vi "interactive_tester.vi"() -> ()   [LabVIEW 2024]
doc: "This VI can perform a measurement with the stimuli set by the Load control.\nBy pressing Update Values the measurement is performed."
uses:
  ctl_loads_enum.ctl
  ctl_stimuli_cluster.ctl
panel:
  out "Vdrop =":dbl
  out "Device OK":bool
  in  "btn_test_device":bool
  in  "DAQmx Device Name":tag="Dev1"
  out "Measurement in progress...":bool
  in  "btn_stop":bool
  in  "btn_update":bool
  out "Pin =":dbl
  out "Iout =":dbl
  in  "Load =":T1=enum."10Ohm"
  out "Efficiency =":dbl
  out "Pout =":dbl
  out "Vout =":dbl
  in  "Rsense =":dbl
  out "Iin =":dbl
  out "Vin =":dbl
  out "RL4":bool=TRUE
  out "RL3":bool=TRUE
  out "RL2":bool=TRUE
  out "RL1":bool=TRUE
  # "V"
  # "A"
  # "9 V"
  # "A"
  # "LM317"
  # "W"
  # "W"
  # "Ohm"
  # "V"
  # "DC-DC converter"
  # "V"
  # "%"
  # "Test the device connection before start measuring"
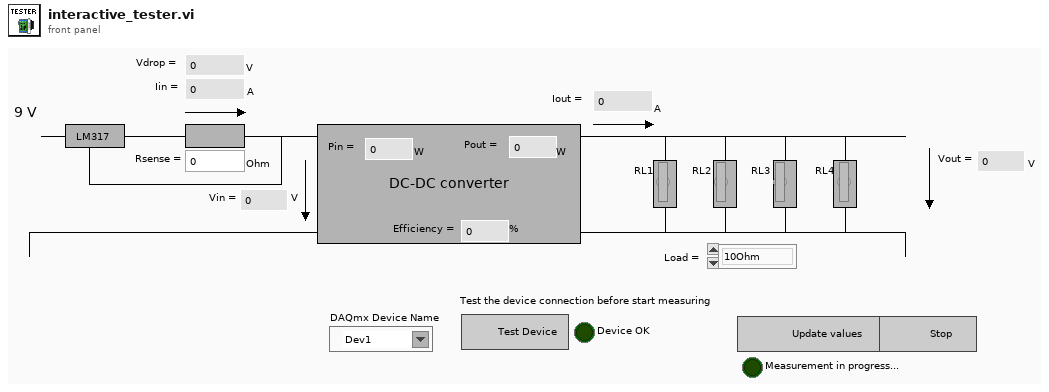
[diagram p1: front panel]
types:
  T1 = typedef "ctl_loads_enum.ctl" = enum16{"NO LOAD", "10Ohm", "6.8Ohm", "4.7Ohm", "3.3Ohm", "2.4Ohm", "1.6Ohm", "1.3Ohm"}
  T2 = typedef "ctl_stimuli_cluster.ctl" = cluster{"Load":T1, "Rsense Value":dbl}
  T3 = typedef "ctl_load_set_cluster.ctl" = cluster{"Resistor 1":bool, "Resistor 2":bool, "Resistor 3":bool, "Resistor 4":bool}
  T4 = typedef "ctl_test_outputs_cluster.ctl" = cluster{"Output V avg":dbl, "Output V ampl":dbl, "Input Current":dbl, "Output Current":dbl, "Efficiency %":dbl, "Input V avg":dbl, "Input Power":dbl, "Output Power":dbl, "Rsense Vdrop":dbl}
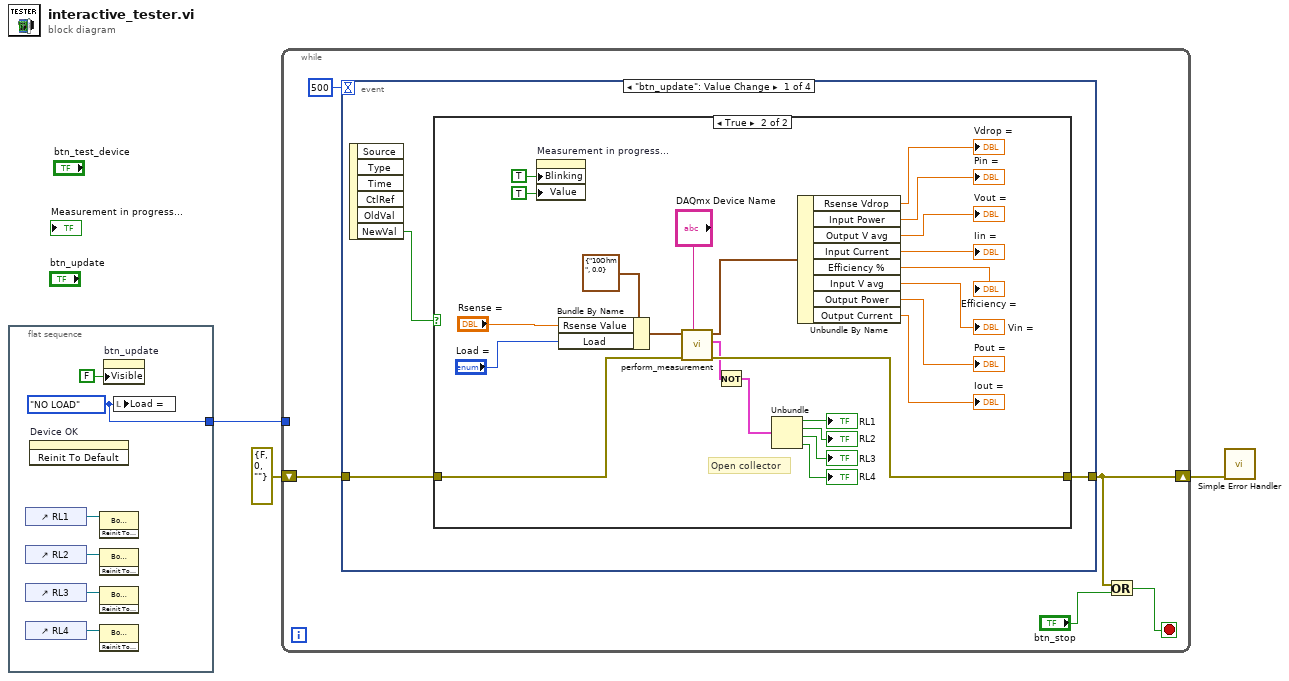
[diagram p0: block diagram]
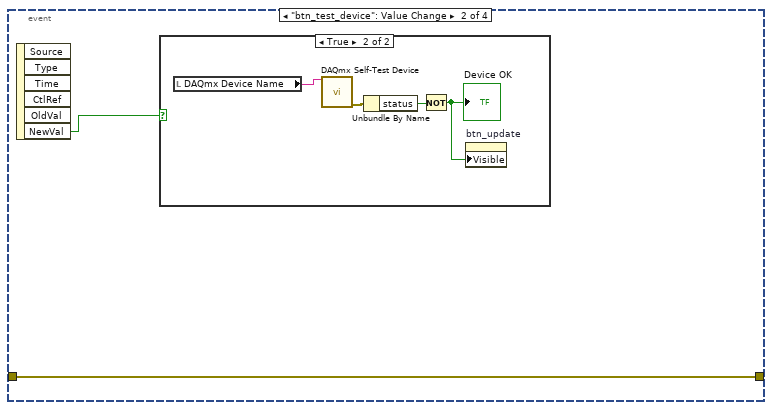
[diagram p3: hidden frame]
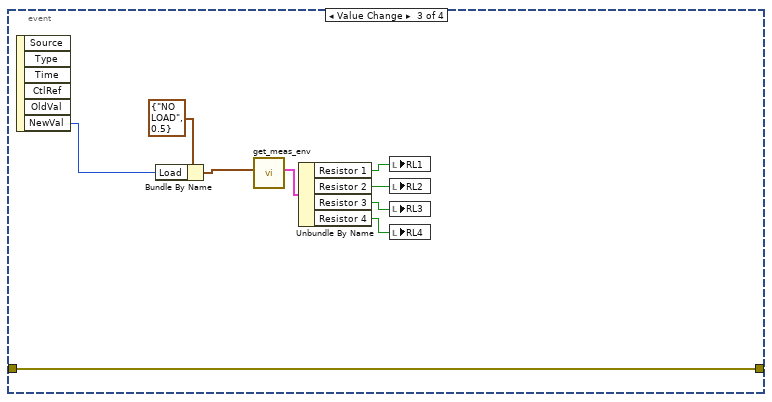
[diagram p5: hidden frame]
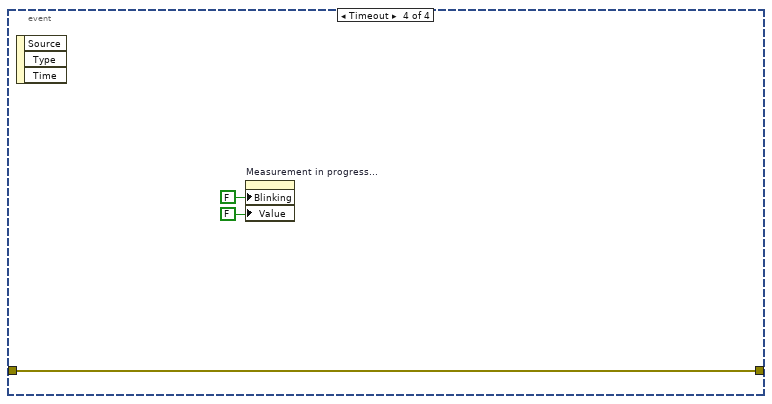
[diagram p6: hidden frame]
diagram:
  n1 = flat-sequence {
    tunnel: [w9] -> w3
    frame #0 {
      w9 = ctl_loads_enum."NO LOAD" ("Load =")
      n2 = control-ref of="RL1"() -> (w7:refnum<vi>)
      n3 = control-ref of="RL2"() -> (w6:refnum<vi>)
      n4 = control-ref of="RL3"() -> (w5:refnum<vi>)
      n5 = control-ref of="RL4"() -> (w4:refnum<vi>)
      n6 = invoke on="Device OK" class="Bool (strict)" method="Reinit To Default"() -> ()  [unwired: 3 in, 3 out]
      n7 = invoke class="Bool (strict)" method="Reinit To Default"(reference=w7) -> ()  [unwired: 2 in, 3 out]
      n8 = invoke class="Bool (strict)" method="Reinit To Default"(reference=w6) -> ()  [unwired: 2 in, 3 out]
      n9 = invoke class="Bool (strict)" method="Reinit To Default"(reference=w5) -> ()  [unwired: 2 in, 3 out]
      n10 = invoke class="Bool (strict)" method="Reinit To Default"(reference=w4) -> ()  [unwired: 2 in, 3 out]
      n11 = property on="btn_update" class="Bool (strict)"("Visible"=FALSE) -> ()  [unwired: 2 in, 2 out]
      n12 = local write "Load ="(w9) -> ()
    }
  }
  n13 = while {
    tunnel: w3 -> [_]
    shift-right: [w11] -> w1
    shift-left: errorcluster {"status"=FALSE, "code"=0, "source"=""} ("error out") -> [w13]
    stop <- w10 stop-if-true
    n14 = event shown="[0] \"btn_update\": Value Change" {
      selector: _ -> [_ _ _ _]
      dyn-events: _ -> [_ _ _ _]
      timeout: 500 -> [_ _ _ _]
      tunnel: [w16 w44 w49 w58] -> w11
      tunnel: w13 -> [w15 w44 w49 w58]
      event "btn_update": Value Change {
        n15 = event-data() -> ("NewVal"=w17:bool)  [unwired: 1 in, 5 out]
        n16 = case shown="True" w17 {
          tunnel: [w18 w24] -> w16
          tunnel: w15 -> [w18 w23]
          frame False {
          }
          frame True {
            # "Open collector"
            n17 = property on="Measurement in progress..." class="Bool (strict)"("Blinking"=TRUE, "Value"=TRUE ("Measurement in progress...")) -> ()  [unwired: 2 in, 2 out]
            n18 = Bundle By Name(cluster=T2 {"Load"=enum."10Ohm", "Rsense Value"=0.0} ("Stimuli"), "Rsense Value"="Rsense =", "Load"="Load =") -> (w39:T2)
            n19 = call "perform_measurement.vi"("DAQmx Device Name"="DAQmx Device Name", "error in"=w23, "Stimuli"=w39) -> ("error out"=w24:errorcluster, "Load Set"=w21:T3, "Outputs"=w34:T4)  [unwired: 6 in]
            n20 = Not(x=w21) -> (.not. x?=w20:T3)
            n21 = Unbundle(w20) -> ("Resistor 1"=→"RL1":bool, "Resistor 2"=→"RL2":bool, "Resistor 3"=→"RL3":bool, "Resistor 4"=→"RL4":bool)
            n22 = Unbundle By Name(w34) -> ("Rsense Vdrop"=→"Vdrop =":dbl, "Input Power"=→"Pin =":dbl, "Output V avg"=→"Vout =":dbl, "Input Current"=→"Iin =":dbl, "Efficiency %"=→"Efficiency =":dbl, "Input V avg"=→"Vin =":dbl, "Output Power"=→"Pout =":dbl, "Output Current"=→"Iout =":dbl)
          }
        }
      }
      event "btn_test_device": Value Change {
        n23 = event-data() -> ("NewVal"=w43:bool)  [unwired: 1 in, 5 out]
        n24 = case shown="True" w43 {
          frame False {
          }
          frame True {
            n25 = local read "DAQmx Device Name"() -> (w48:tag)
            n26 = call <vilib>:"DAQmx Self-Test Device.vi"("device in"=w48) -> ("error out"=w47:errorcluster)  [unwired: 14 in]
            n27 = Unbundle By Name(w47) -> ("status"=w46:bool)
            n28 = Not(x=w46) -> (.not. x?=w45:bool)
            "Device OK" <- w45
            n29 = property on="btn_update" class="Bool (strict)"("Visible"=w45) -> ()  [unwired: 2 in, 2 out]
          }
        }
      }
      event Value Change {
        n30 = event-data() -> ("NewVal"=w50:T1)  [unwired: 1 in, 5 out]
        n31 = Bundle By Name(cluster=T2 {"Load"=enum."NO LOAD", "Rsense Value"=0.5} ("Stimuli"), "Load"=w50) -> (w56:T2)
        n32 = call "get_meas_env.vi"("Stimuli"=w56) -> ("Load Set"=w55:T3)  [unwired: 9 in, 1 out]
        n33 = Unbundle By Name(w55) -> ("Resistor 1"=w54:bool, "Resistor 2"=w53:bool, "Resistor 3"=w52:bool, "Resistor 4"=w51:bool)
        n34 = local write "RL1"(w54) -> ()
        n35 = local write "RL2"(w53) -> ()
        n36 = local write "RL3"(w52) -> ()
        n37 = local write "RL4"(w51) -> ()
      }
      event Timeout {
        n38 = event-data() -> ()  [unwired: 1 in, 3 out]
        n39 = property on="Measurement in progress..." class="Bool (strict)"("Blinking"=FALSE, "Value"=FALSE ("Measurement in progress...")) -> ()  [unwired: 2 in, 2 out]
      }
    }
    n40 = Or(x=w11, y="btn_stop") -> (x .or. y?=w10:bool)
  }
  n41 = call <vilib>:"Simple Error Handler.vi"("error in (no error)"=w1) -> ()  [unwired: 4 in, 5 out]
